vi "Log State Type.vi"(9 "Complete? (T)/Start(F)":bool, 10 "Source Module":string, 11 "‘State":string) -> (3 "CSM_GlobalLog_STATE_TYPE":T1)   [LabVIEW 2017, in "Communicable State Machine.lvlib" / "LogFilter.lvclass"]
doc: "### Log State Type.vi\n\n-- <b>Controls</b> --\n- <b>Complete(T)/Start(F)</b>:\n- <b>Source Module</b>:\n- <b>State</b>:\n\n-- <b>Indicators</b> --\n- <b>CSM_GlobalLog_STATE_TYPE</b>:"
uses:
  LogFilter.lvclass
  Typedef/_CSM_GlobalLog_STATE_TYPE.ctl
  Communicable State Machine.lvlib
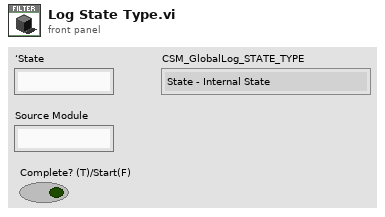
[diagram p1: front panel]
types:
  T1 = typedef "Communicable State Machine.lvlib/_CSM_GlobalLog_STATE_TYPE.ctl" = enum16{"State - Internal State", "State - External Message", "State - Response", "State - Complete"}
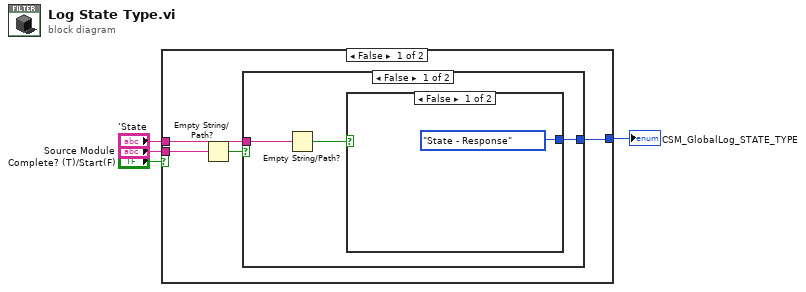
[diagram p0: block diagram]
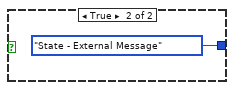
[diagram p2: hidden frame]
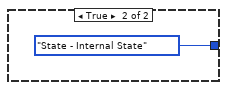
[diagram p3: hidden frame]
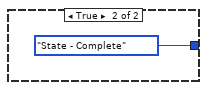
[diagram p4: hidden frame]
diagram:
  n1 = case shown="False" "Complete? (T)/Start(F)" {
    tunnel: "Source Module" -> [w8 _]
    tunnel: "‘State" -> [w6 _]
    tunnel: [w5 _CSM_GlobalLog_STATE_TYPE."State - Complete" ("CSM_GlobalLog_STATE_TYPE")] -> w4
    frame False {
      n2 = Empty String/Path?(string/path=w8) -> (empty?=w7:bool)
      n3 = case shown="False" w7 {
        tunnel: w6 -> [w11 _]
        tunnel: [w9 _CSM_GlobalLog_STATE_TYPE."State - Internal State" ("CSM_GlobalLog_STATE_TYPE")] -> w5
        frame False {
          n4 = Empty String/Path?(string/path=w11) -> (empty?=w10:bool)
          n5 = case shown="False" w10 {
            tunnel: [_CSM_GlobalLog_STATE_TYPE."State - Response" ("CSM_GlobalLog_STATE_TYPE") _CSM_GlobalLog_STATE_TYPE."State - External Message" ("CSM_GlobalLog_STATE_TYPE")] -> w9
            frame False {
            }
            frame True {
            }
          }
        }
        frame True {
        }
      }
    }
    frame True {
    }
  }
  "CSM_GlobalLog_STATE_TYPE" <- w4
